vi "Get Channel Units From Section by #.vi"(7 "Section name":string, 8 "error in (no error)":errorcluster, 10 "CH#":i32, 11 "Item Ref in":T1 format="%.0x") -> (0 "error out":errorcluster, 2 "Units":string, 3 "Item Ref out":T1 format="%.0x")   [LabVIEW 2023, in "NI 272x Resistive Simulation Custom Device Configuration.lvlib"]
uses:
  NI 272x Resistive Simulation Custom Device Configuration.lvlib
  <vilib>/NI VeriStand/Custom Device API/Custom Device Item Ref.ctl
  <vilib>/NI VeriStand/Custom Device API/Custom Device API.lvlib
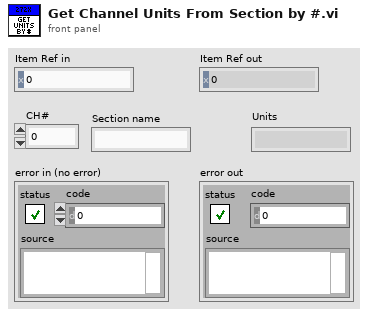
[diagram p1: front panel]
types:
  T1 = typedef "Custom Device API.lvlib/Custom Device Item Ref.ctl" = u64
  T2 = typedef "Custom Device API.lvlib/Custom Device Channel.ctl" = cluster{"Type":T3, "Units":string, "Default Value":dbl, "Faultable":bool, "Scalable":bool}
  T3 = typedef "Custom Device API.lvlib/Custom Device Channel Type.ctl" = enum16{"Input", "Output"}
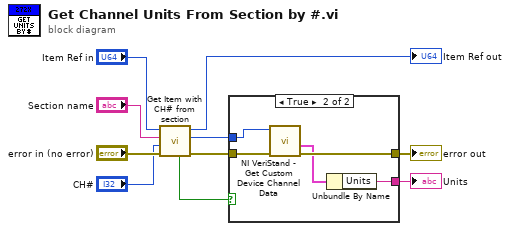
[diagram p0: block diagram]
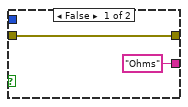
[diagram p2: hidden frame]
diagram:
  n1 = call "Get Item with CH# from section.vi"("error in (no error)"="error in (no error)", "CH#"="CH#", "Section containing ch#"="Section name", "Item Ref in"="Item Ref in") -> ("error out"=w5:errorcluster, "Matching CH# item in Specified Section"=w8:T1, "Item Ref out"=→"Item Ref out":T1, "Found"=w1:bool)  [unwired: 4 in]
  n2 = case shown="True" w1 {
    tunnel: w8 -> [_ w17]
    tunnel: [w11 w16] -> w10
    tunnel: w5 -> [w11 w15]
    tunnel: ["Ohms" ("Units") w13] -> w3
    frame False {
    }
    frame True {
      n3 = call <vilib>:"NI VeriStand - Get Custom Device Channel Data.vi"("error in (no error)"=w15, "Channel Ref in"=w17) -> ("error out"=w16:errorcluster, "Channel"=w14:T2)  [unwired: 4 in, 4 out]
      n4 = Unbundle By Name(w14) -> ("Units"=w13:string)
    }
  }
  "error out" <- w10
  "Units" <- w3
